vi "MoveLeft.vi"(0 "Grids In":i32[][](array[numeric])) -> (1 "Grid Out":i32[][](array[numeric]), 2 "Score":i32, 3 "Moved?":bool)   [LabVIEW 2018]
doc: "Move grids left."
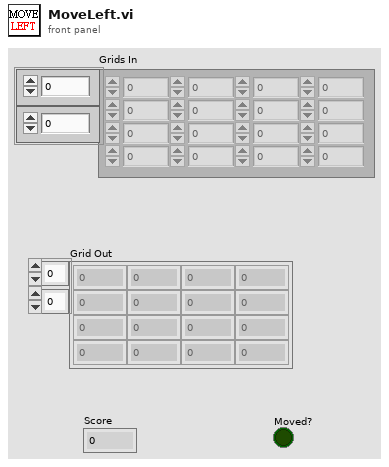
[diagram p1: front panel]
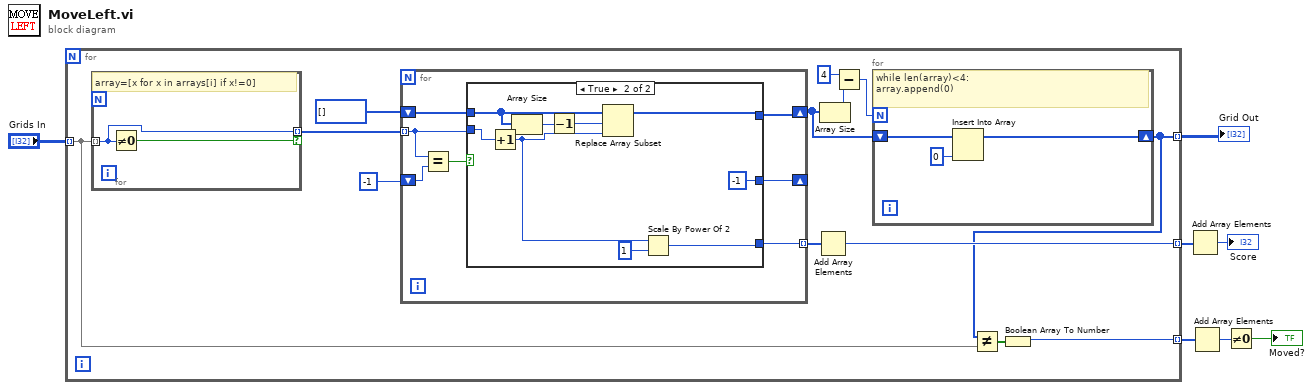
[diagram p0: block diagram]
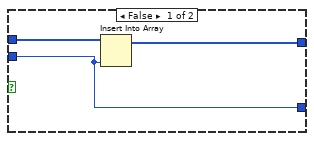
[diagram p2: hidden frame]
diagram:
  n1 = for {
    tunnel: "Grids In" -> [w10] mode=indexing
    tunnel: [w16] -> w7 mode=indexing
    tunnel: [w11] -> w5 mode=indexing
    tunnel: [w8] -> w3 mode=indexing
    n2 = for {
      tunnel: w10 -> [w44] mode=indexing
      tunnel: [w44] -> w20 mode=indexing if=w43
      # "array=[x for x in arrays[i] if x!=0]"
      n3 = Not Equal To 0?(x=w44) -> (x != 0?=w43:bool)
    }
    n4 = for {
      shift-right: [w26] -> w12
      shift-left: i32[] [] -> [w28]
      tunnel: w20 -> [w27] mode=indexing
      shift-right: [w25] -> _
      shift-left: -1 -> [w30]
      tunnel: [w24] -> w17 mode=indexing
      n5 = Equal?(x=w27, y=w30) -> (x = y?=w29:bool)
      n6 = case shown="True" w29 {
        tunnel: w28 -> [w33 w38]
        tunnel: w27 -> [w31 w41]
        tunnel: [w32 w40] -> w26
        tunnel: [w31 -1 ("Numeric")] -> w25
        tunnel: [_ w34] -> w24
        frame False {
          n7 = Insert Into Array(array=w33, new element=w31) -> (w32:i32[])  [unwired: 1 in]
        }
        frame True {
          n8 = Increment(x=w41) -> (x+1=w36:i32)
          n9 = Array Size(array=w38) -> (size(s)=w42:i32)
          n10 = Decrement(x=w42) -> (x-1=w37:i32)
          n11 = Replace Array Subset(array=w38, new element=w36, index=w37) -> (w40:i32[])
          n12 = Scale By Power Of 2(n=w36, x=1) -> (x*2^n=w34:i32)
        }
      }
    }
    n13 = Add Array Elements(numeric array=w17) -> (sum=w16:i32)
    n14 = Array Size(array=w12) -> (size(s)=w15:i32)
    n15 = Subtract(x=4, y=w15) -> (x-y=w14:i32)
    n16 = for {
      N: w14 -> [_]
      shift-right: [w21] -> w11
      shift-left: w12 -> [w23]
      # "while len(array)<4:\narray.append(0)"
      n17 = Insert Into Array(array=w23, new element=0 ("new element/subarray")) -> (w21:i32[])  [unwired: 1 in]
    }
    n18 = Not Equal?(x=w11, y=w10) -> (x != y?=w9:bool[])
    n19 = Boolean Array To Number(Boolean array=w9) -> (number=w8:u32)
  }
  "Grid Out" <- w5
  n20 = Add Array Elements(numeric array=w7) -> (sum=→"Score":i32)
  n21 = Add Array Elements(numeric array=w3) -> (sum=w2:u32)
  n22 = Not Equal To 0?(x=w2) -> (x != 0?=→"Moved?":bool)
